vi "SRV_Init_TCP Comm.vi"(8 "error in (no error)":errorcluster, 11 "SRV IP Address":string) -> (0 "error out":errorcluster, 2 "SRV IP Address dup":string, 3 "connection ID":refnum<k5>)   [LabVIEW 2009]
doc: "Opens a session with the SRV.\n\n\nWritten for Benilde St. Margaret's School - Tim Jump\nBy Doug Schmertman - Logic PD\nCopyright 2012"
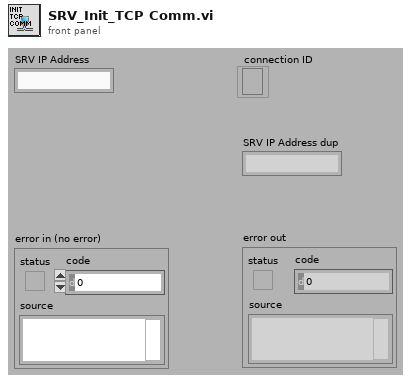
[diagram p1: front panel]
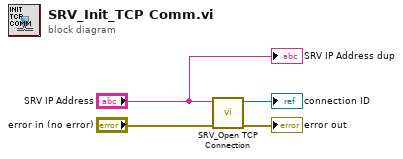
[diagram p0: block diagram]
diagram:
  n1 = call "SRV_Open TCP Connection.vi"("error in (no error)"="error in (no error)", "IP address"="SRV IP Address") -> ("error out"=→"error out":errorcluster, "connection ID"=→"connection ID":refnum<k5>)  [unwired: 8 in]
  "SRV IP Address dup" <- "SRV IP Address"
